vi "信息接收.vi"() -> ()   [LabVIEW 2016, in "环境动力监测库.lvlib" / "NMEA.lvlib"]
uses:
  NMEA.lvlib
  <vilib>/Instr/_visa.llb/VISA Configure Serial Port (Instr).vi
panel:
  out "匹配之前的子字符串 2":string
  out "匹配之前的子字符串":string
  out "read buffer":string
  in  "停止":bool
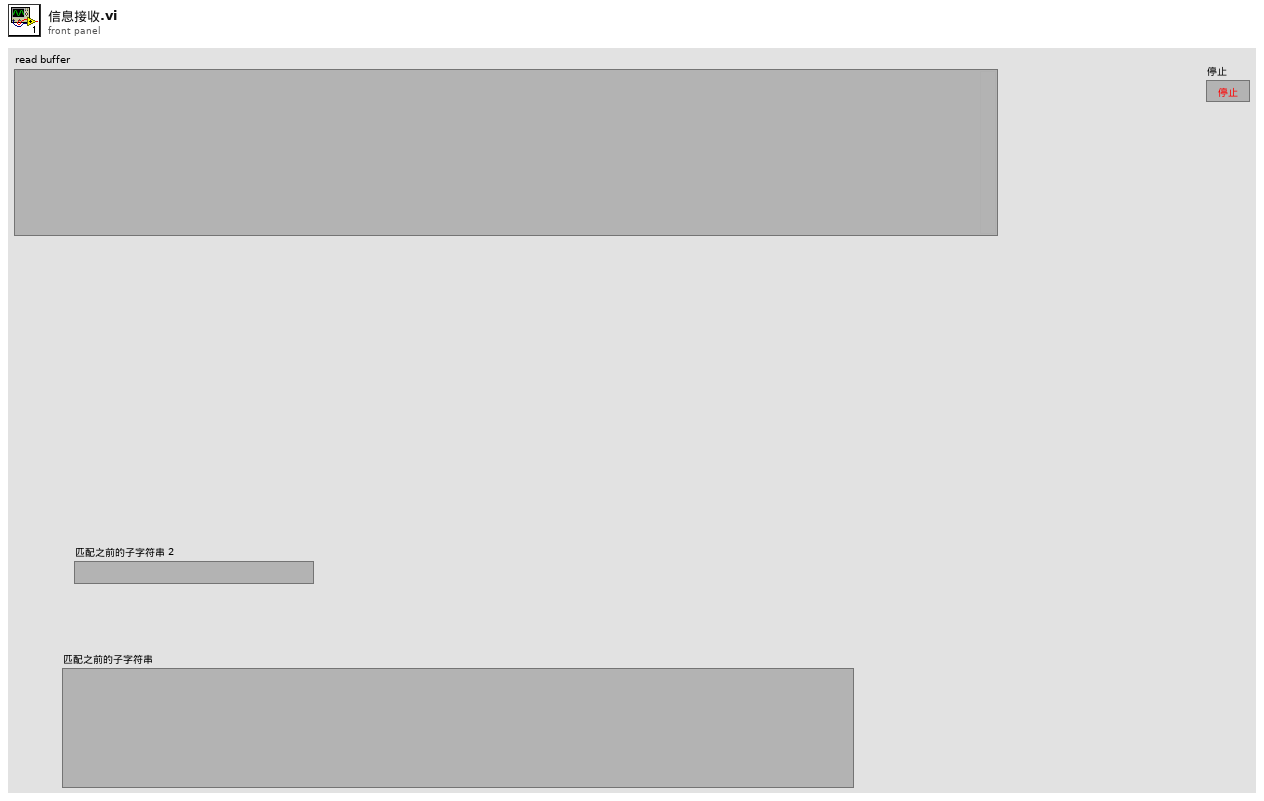
[diagram p1: front panel]
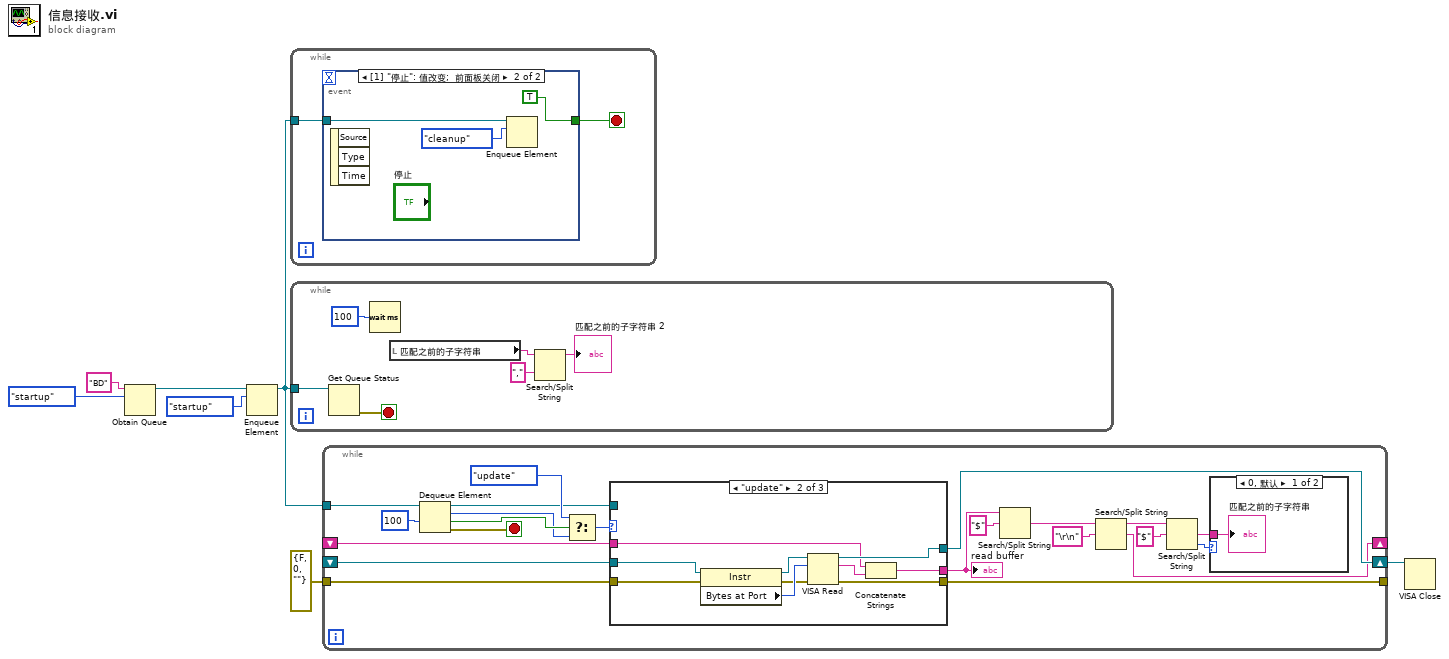
[diagram p0: block diagram]
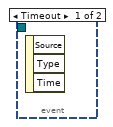
[diagram p2: hidden frame]
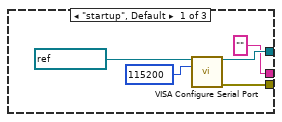
[diagram p4: hidden frame]
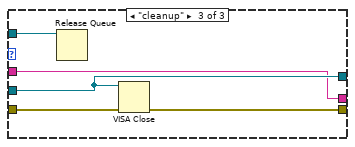
[diagram p5: hidden frame]
diagram:
  n1 = Obtain Queue(name (unnamed)="BD" ("名称（未命名）"), element data type=enum16{"startup", "update", "cleanup"}."startup" ("枚举")) -> (queue out=w4:refnum<queue>)  [unwired: 3 in, 2 out]
  n2 = Enqueue Element(queue=w4, element=enum16{"startup", "update", "cleanup"}."startup" ("元素")) -> (queue out=w2:refnum<queue>)  [unwired: 2 in, 2 out]
  n3 = while {
    tunnel: w2 -> [w9]
    stop <- w8 stop-if-true
    n4 = event shown="[1] \"停止\": 值改变;  前面板关闭" {
      selector: _ -> [_ _]
      dyn-events: _ -> [_ _]
      timeout: _ -> [_ _]
      tunnel: w9 -> [_ w12]
      tunnel: [_ TRUE] -> w8
      event Timeout {
        n5 = event-data() -> ()  [unwired: 1 in, 3 out]
      }
      event "停止": Value Change; Panel Close {
        n6 = event-data() -> ()  [unwired: 1 in, 3 out]
        n7 = Enqueue Element(queue=w12, element=enum16{"startup", "update", "cleanup"}."cleanup" ("元素")) -> ()  [unwired: 2 in, 3 out]
      }
    }
  }
  n8 = while {
    tunnel: w2 -> [w18]
    stop <- w17 stop-if-true
    n9 = Get Queue Status(queue=w18) -> (error out=w17:errorcluster)  [unwired: 2 in, 7 out]
    n10 = Wait (ms)(milliseconds to wait=u32 100 ("等待时间（毫秒）")) -> ()  [unwired: 1 out]
    n11 = local read "匹配之前的子字符串"() -> (w15:string)
    n12 = Search/Split String(string=w15, search string/char (-)="," ("搜索字符串/字符(-)")) -> (substring before match=→"匹配之前的子字符串 2":string)  [unwired: 1 in, 2 out]
  }
  n13 = while {
    shift-right: [w39] -> w5
    shift-left: _ -> [w38]
    shift-right: [w23] -> _
    shift-left: _ -> [w36]
    tunnel: w2 -> [w35]
    tunnel: errorcluster {"status"=FALSE, "code"=0, "source"=""} ("error out") -> [w37]
    tunnel: [w40] -> _
    stop <- w29 stop-if-true
    n14 = Dequeue Element(queue=w35, timeout in ms (-1)=100 ("超时毫秒(-1)")) -> (queue out=w28:refnum<queue>, element=w31:enum16{"startup", "update", "cleanup"}, timed out?=w33:bool, error out=w29:errorcluster)  [unwired: 1 in]
    n15 = Select(t=enum16{"startup", "update", "cleanup"}."update" ("枚举"), s=w33, f=w31) -> (s? t:f=w30:enum16{"startup", "update", "cleanup"})
    n16 = case shown="\"update\"" w30 {
      tunnel: [w43 w47 w60] -> w40
      tunnel: [w44 w53 w59] -> w39
      tunnel: w38 -> [_ w56 w59]
      tunnel: ["" ("read buffer") w50 w58] -> w24
      tunnel: w37 -> [_ w49 w61]
      tunnel: w36 -> [_ w52 w58]
      tunnel: w28 -> [_ _ w57]
      frame "startup", Default {
        n17 = call-poly "VISA Configure Serial Port"("VISA resource name"=refnum<visa-resource-name> "COM17", "baud rate (9600)"=u32 115200) -> ("VISA resource name out"=w44:refnum<visa-resource-name>, "error out"=w43:errorcluster)  [unwired: 12 in]
      }
      frame "update" {
        n18 = property class="Instr"(reference=w56, error in=w49) -> (reference out=w55:refnum<visa-resource-name>, error out=w48:errorcluster, "Bytes at Port"=w54:u32)
        n19 = VISA Read(VISA resource name=w55, byte count=w54, error in (no error)=w48) -> (VISA resource name out=w53:refnum<visa-resource-name>, read buffer=w51:string, error out=w47:errorcluster)  [unwired: 1 out]
        n20 = Concatenate Strings(w52, w51) -> (w50:string)
      }
      frame "cleanup" {
        n21 = Release Queue(queue=w57) -> ()  [unwired: 2 in, 3 out]
        n22 = VISA Close(VISA resource name=w59, error in (no error)=w61) -> (error out=w60:errorcluster)
      }
    }
    "read buffer" <- w24
    n23 = Search/Split String(string=w24, search string/char (-)="$" ("正则表达式")) -> (match + rest of string=w26:string)  [unwired: 1 in, 2 out]
    n24 = Search/Split String(string=w26, search string/char (-)="\r\n" ("搜索字符串/字符(-)")) -> (substring before match=w21:string, match + rest of string=w23:string)  [unwired: 1 in, 1 out]
    n25 = Search/Split String(string=w21, search string/char (-)="$" ("正则表达式")) -> (match + rest of string=w19:string, offset of match=w20:i32)  [unwired: 1 in, 1 out]
    n26 = case shown="0, 默认" w20 {
      tunnel: w19 -> [w41 _]
      frame 0, Default {
        "匹配之前的子字符串" <- w41
      }
      frame -1 {
      }
    }
  }
  n27 = VISA Close(VISA resource name=w5) -> ()  [unwired: 1 in, 1 out]
